vi "Lightfield Software.vi"() -> ()   [LabVIEW 2015]
doc: "Use this template to build a producer/consumer design pattern. Use this template when you need to execute a process, such as data analysis, when a data source, such as a triggered acquisition, produces data at an uneven rate and you need to execute the process when the data becomes available."
uses:
  etc/Other/Backups/Lightfield/Add-in and Automation SDK/Samples/LabVIEW Automation/lightfield-automation-labview/LightField Automation.lvclass
  <vilib>/Utility/file.llb/Write Delimited Spreadsheet (DBL).vi
  Documents/test/SDK 1.2.4 Installer/SDK 1.2.4 Installer/examples/Labview/win64/PE_Filter_SDK/PE_Filter_SDK.lvlib
panel:
  out "PLE total count":dbl
  out "LLTF error":errorcluster
  out "LLTF port":u32
  out "y_Count":dbl
  out "x_Count":dbl
  out "Time-counting":dbl
  in  "?":T1(tab)
  in  "PLE start":bool
  in  "PLE Pause":bool
  in  "PLE save":bool
  out "Min Wavelength":dbl
  out "Max Wavelength":dbl
  out "Current system":string
  out "PLE spectrum":dbl[][](graph)
  in  "Laser WL (nm)":dbl=450.0
  in  "Start WL":dbl=450.0
  in  "End WL":dbl=600.0
  in  "Step (nm)":dbl=1.0
  out "Current WL":dbl=450.0
  in  "Laser WL offset (nm)":dbl=-0.8
  in  "PLE_Autoscale intensity":bool
  in  "2D map_save":bool
  in  "2D map":bool
  in  "Step (um)":dbl=1.0
  in  "x_width (um)":dbl=10.0
  in  "y_width (um)":dbl=10.0
  out "Total Count":dbl
  in  "2D Pause":bool
  out "Cur_pos_x":dbl
  out "Cur_pos_y":dbl
  out "map_plot":dbl[][](graph)
  in  "WL Slide":cluster{dbl, dbl}(slide)={0.0, 1.4141414141414141} scale=700.8419246652234..738.7930212756685
  out "WL":dbl[](array[numeric])
  out "i_max":dbl
  out "i_min":dbl
  in  "Until when (s)":dbl=1.0 caption="Time Target (s)"
  in  "Time-series":bool
  out "Time-series graph":dbl[][](graph)
  in  "Times Pause":bool
  in  "Time Interval (s)":dbl=1.0 caption="Time Target (s)"
  in  "Time-series save":bool
  out "Runging time (s)":dbl
  out "map_data":dbl[][][](array[numeric])
  out "E727 error":errorcluster
  out "Min_y":dbl
  out "Min_x":dbl
  out "Max_y":dbl
  out "Max_x":dbl
  out "E727 Axes":string[](array[string])
  in  "USB settings":cluster{"S/N":string, "USB Search?":bool}={"S/N"="", "USB Search?"=TRUE}
  in  "E727":i32=1 min=1 step=1
  in  "Exposure Time (ms)":dbl=300.0
  in  "Centre WL (nm)":dbl=500.0
  out "Pixel Information":dbl[][](graph)
  in  "ROI":i32=1
  out "PL spectrum":T2(graph)
  out "LightField":refnum<class "LightField Automation.lvclass">
  in  "Experiment name":string="Exp"
  out "error out":errorcluster
  in  "Load":bool
  in  "Single Acquire":bool
  in  "stop":bool
  # "*If you selected \"Full sensor, Binned mode\" in ROI option at LightField, input \"1\""
  # "LLTF Control"
  # "LLTF Information"
  # "* The laser wavelength emitted from the LLTF is off-calibrated by around \"+0.8 nm\".\n* When you save the PLE data, All of the laser wavelength elements will be automatically added around [Laser WL offset \"+0.8 nm\"]."
  # "* Maximum of width is 100 um"
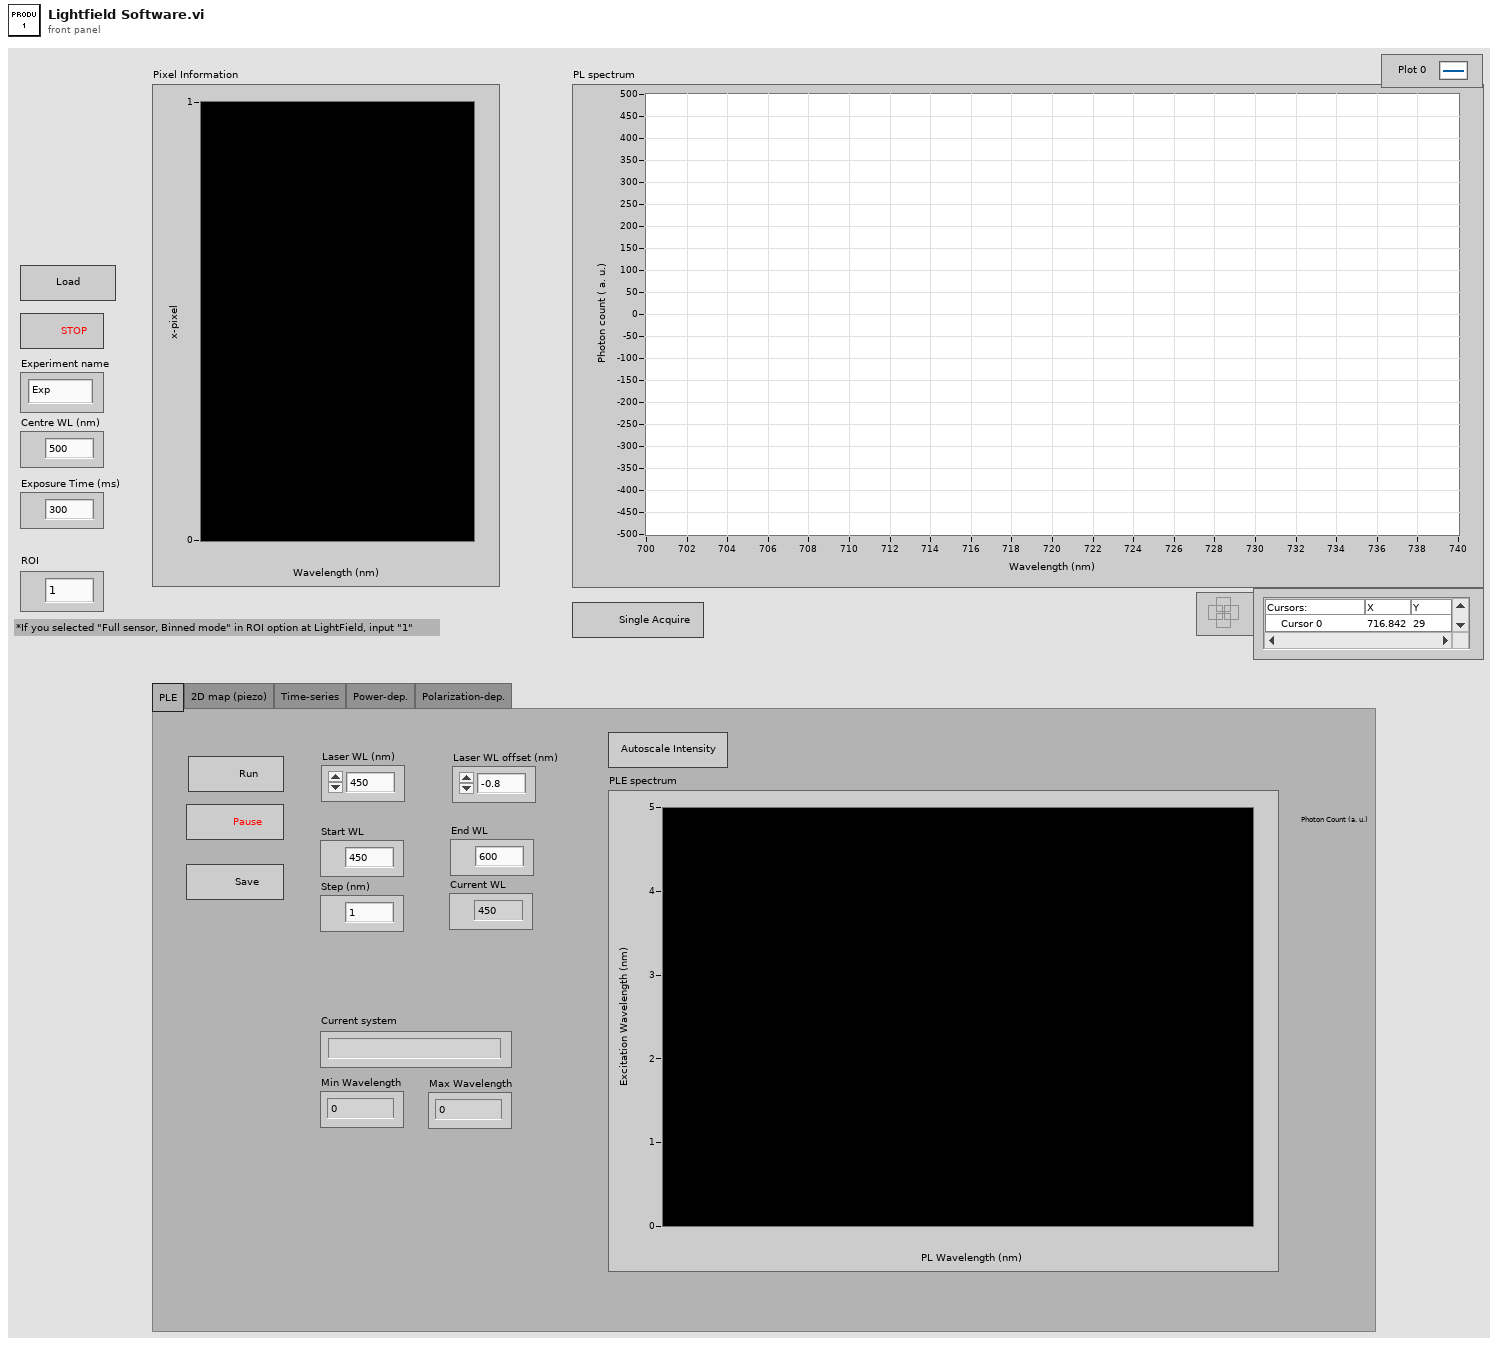
[diagram p1: front panel]
types:
  T1 = enum32{"PLE", "2D map (piezo)", "Time-series", "Power-dep.", "Polarization-dep."}
  T2 = cluster{"ColumnCalibration":dbl[], "ROI 1, Frame 1, Row 1":dbl[]}
  T3 = cluster{"Image":dbl[][][], "Frame Size":cluster{"F":i32, "Y":i32, "X":i32}}[]
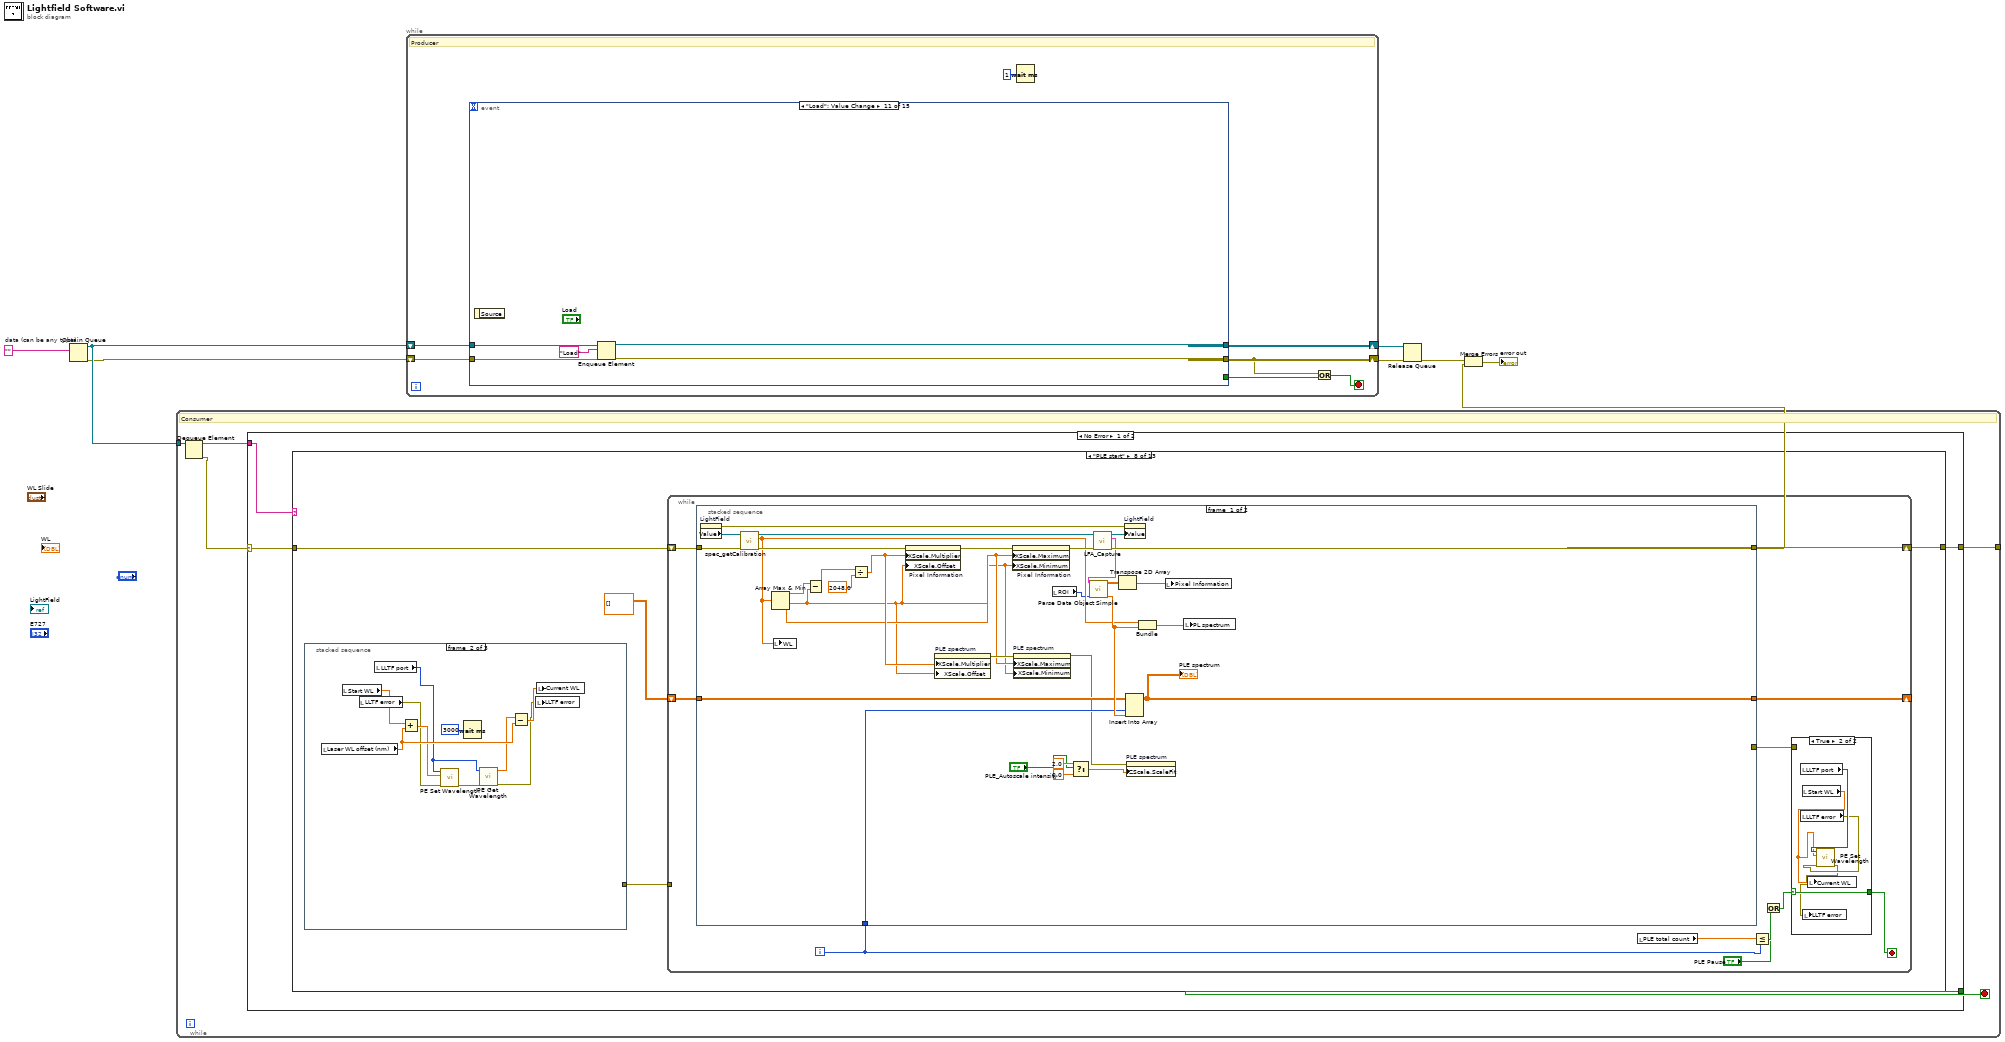
[diagram p0: block diagram]
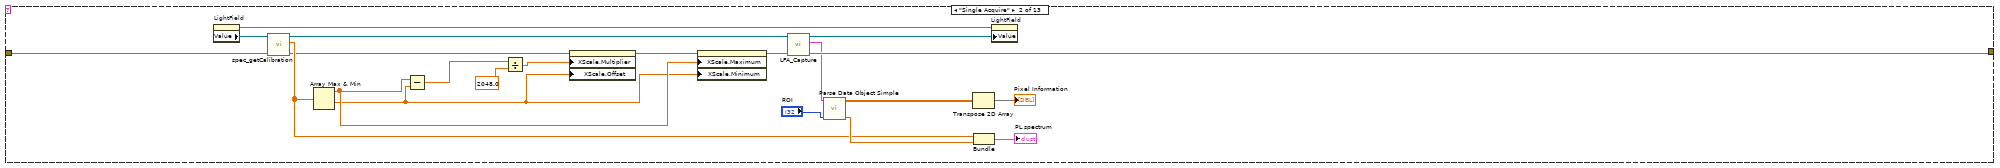
[diagram p3: hidden frame]
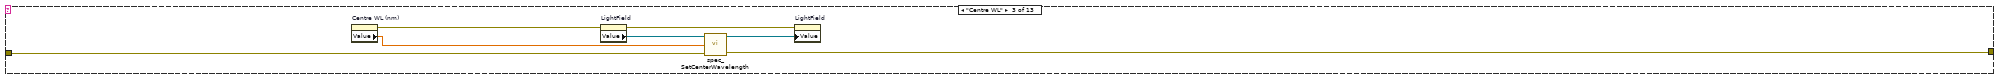
[diagram p4: hidden frame]
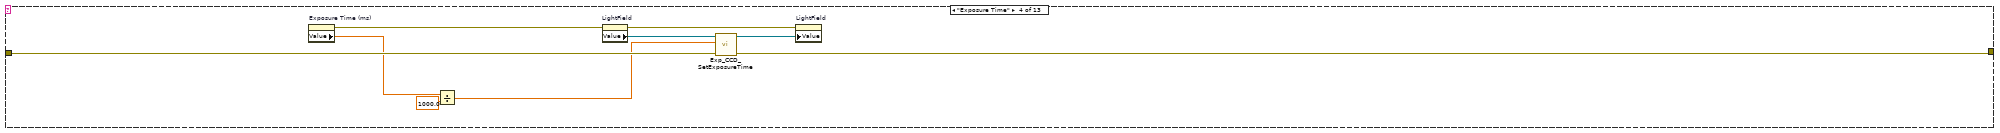
[diagram p5: hidden frame]
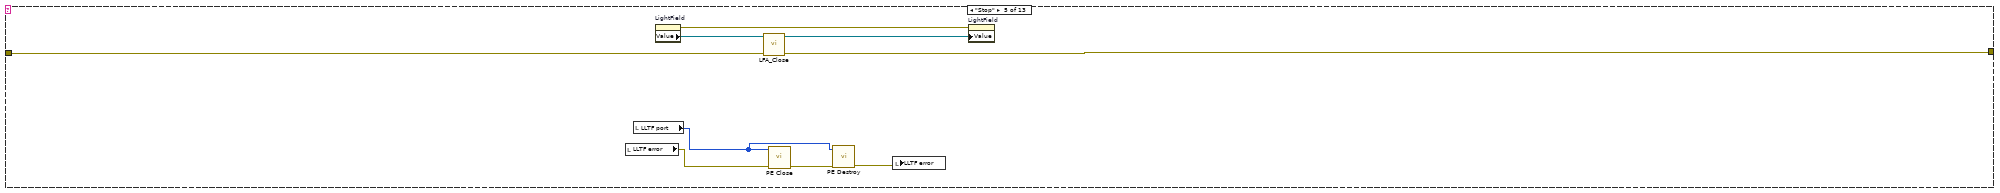
[diagram p6: hidden frame]
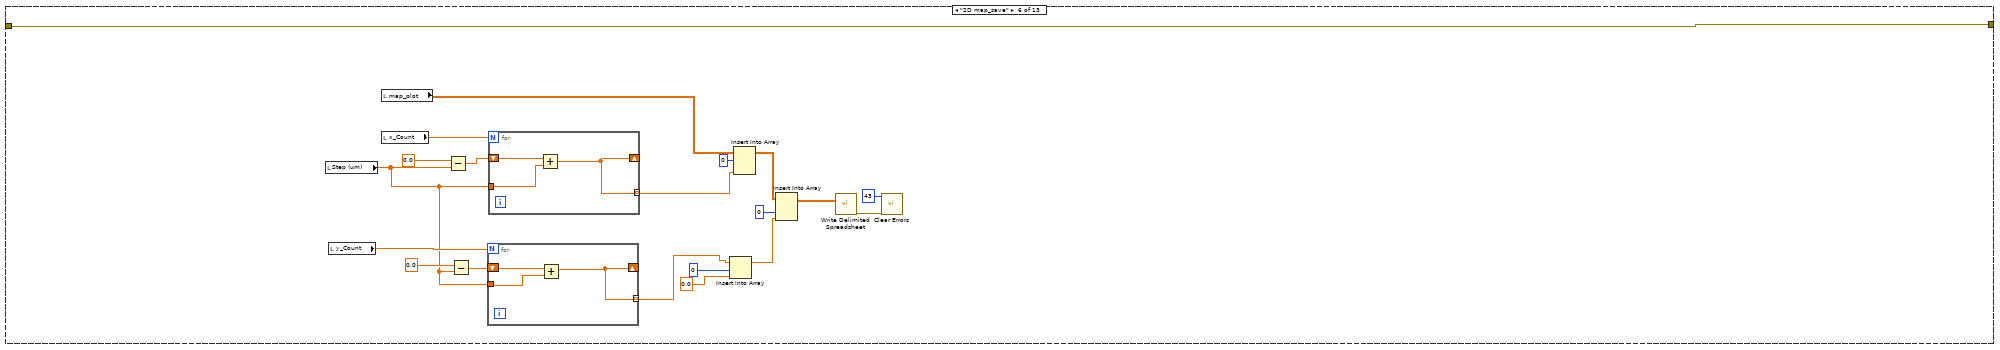
[diagram p7: hidden frame]
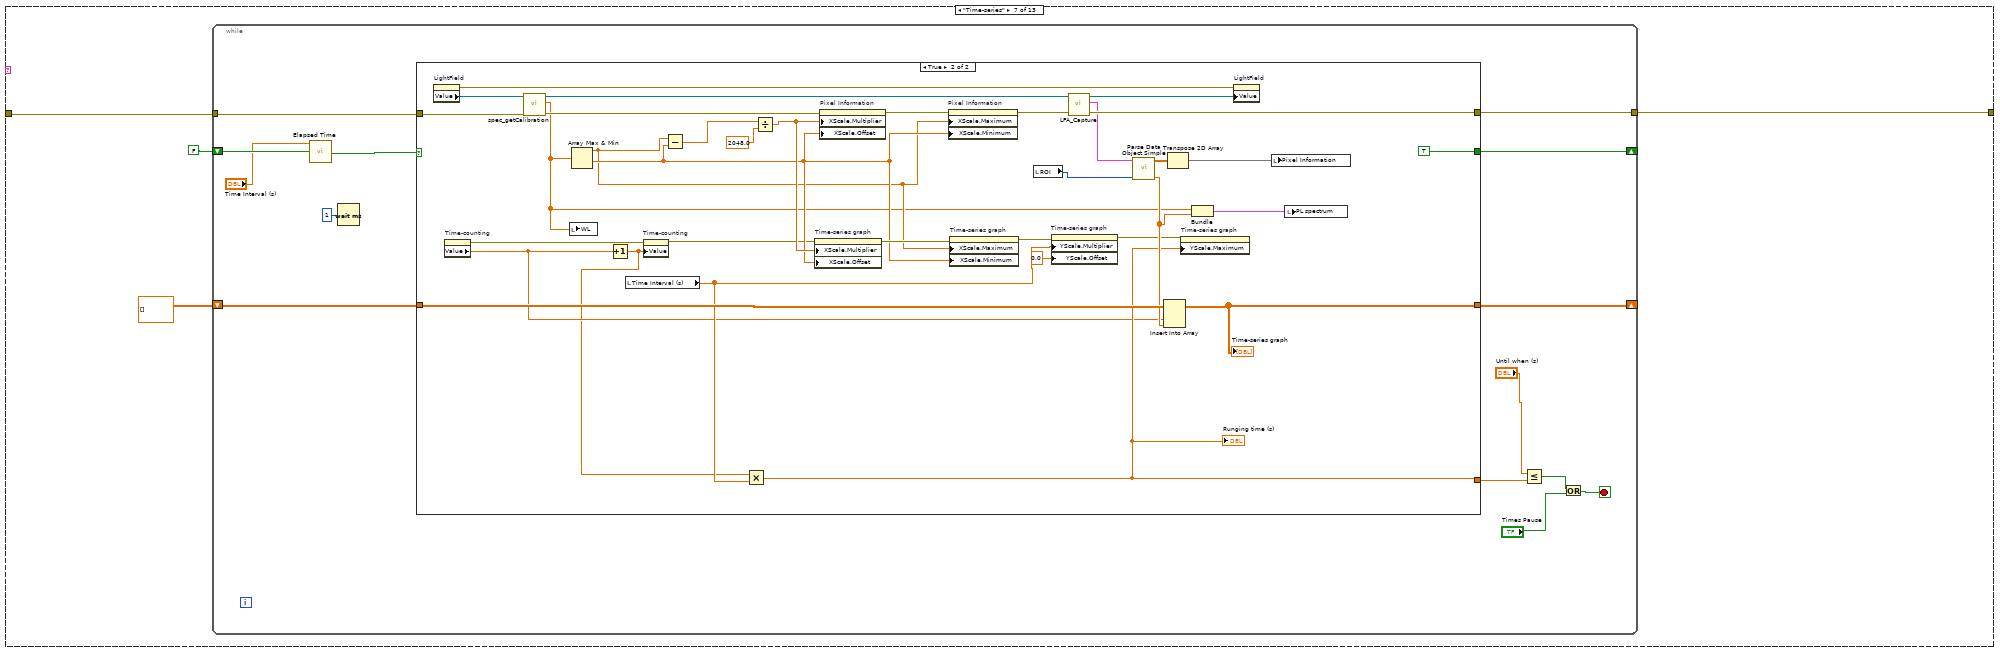
[diagram p8: hidden frame]
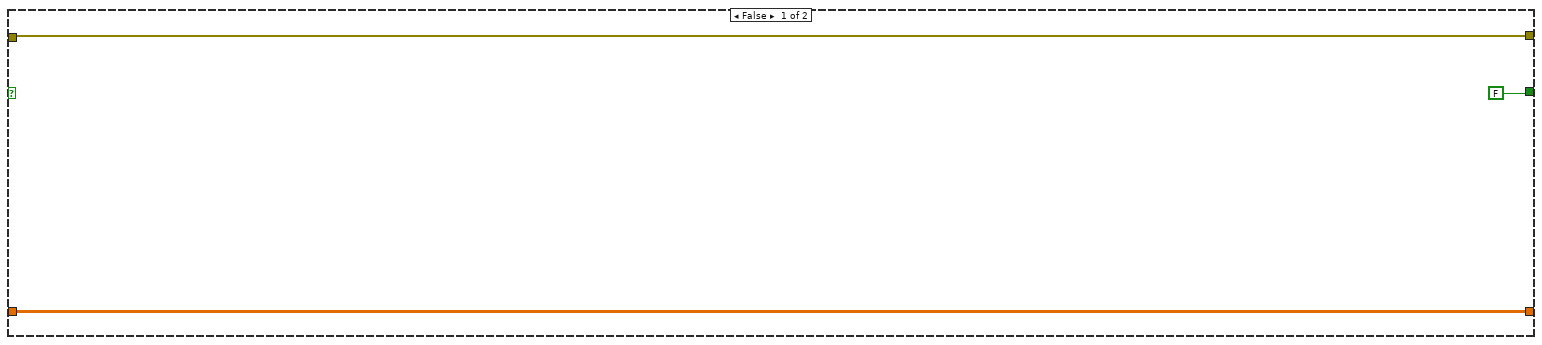
[diagram p9: hidden frame]
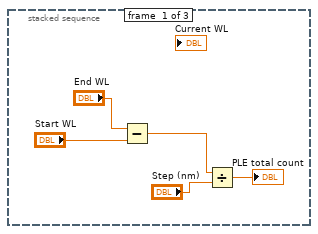
[diagram p10: hidden frame]
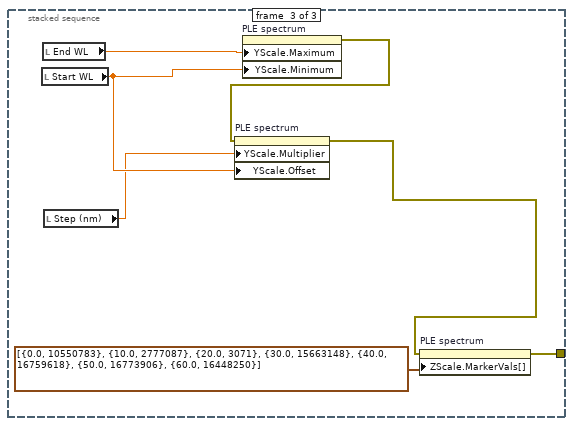
[diagram p11: hidden frame]
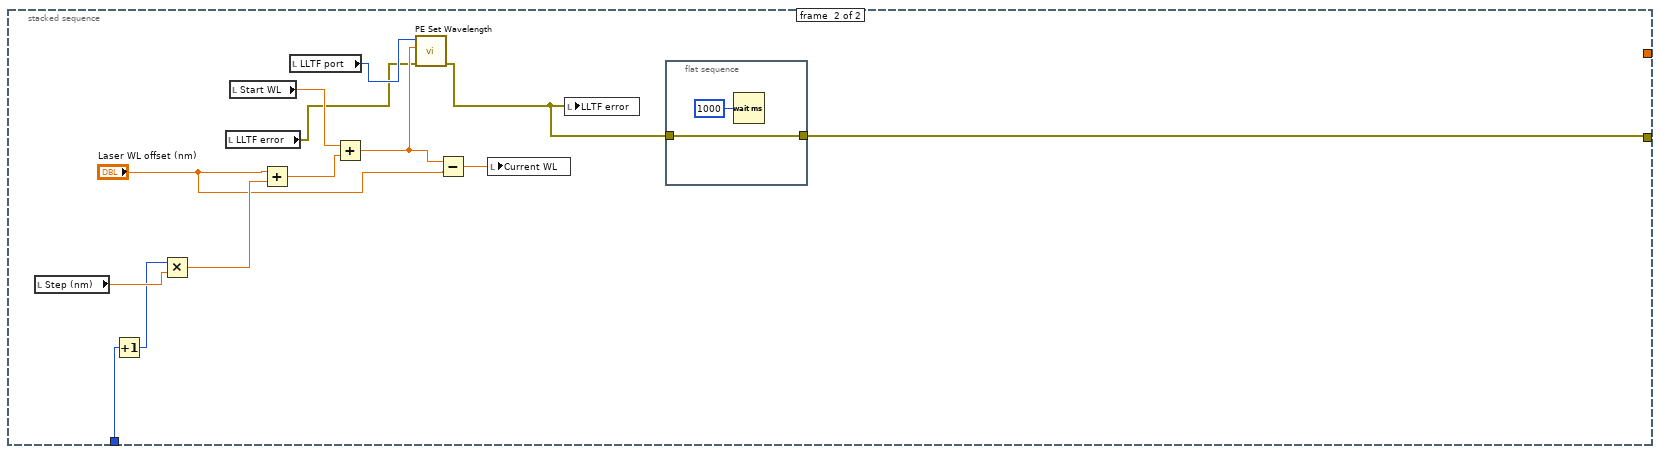
[diagram p13: hidden frame]
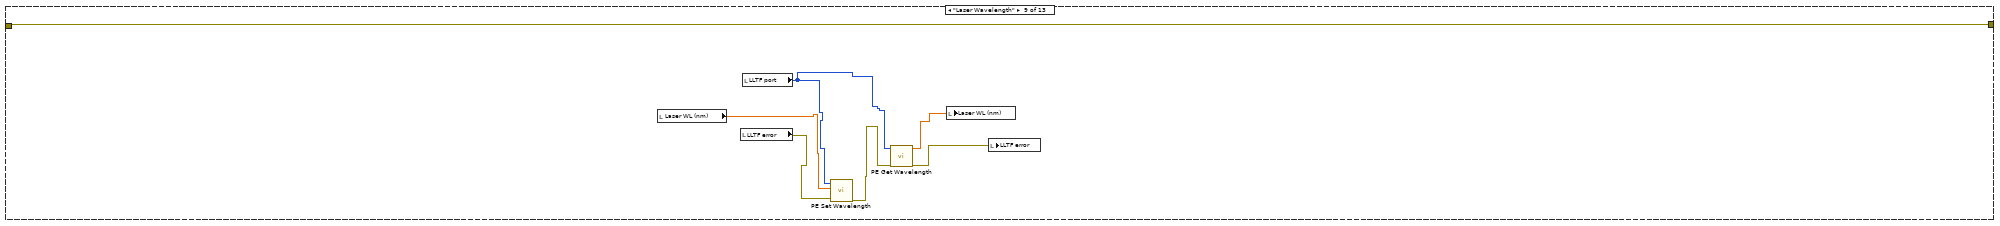
[diagram p14: hidden frame]
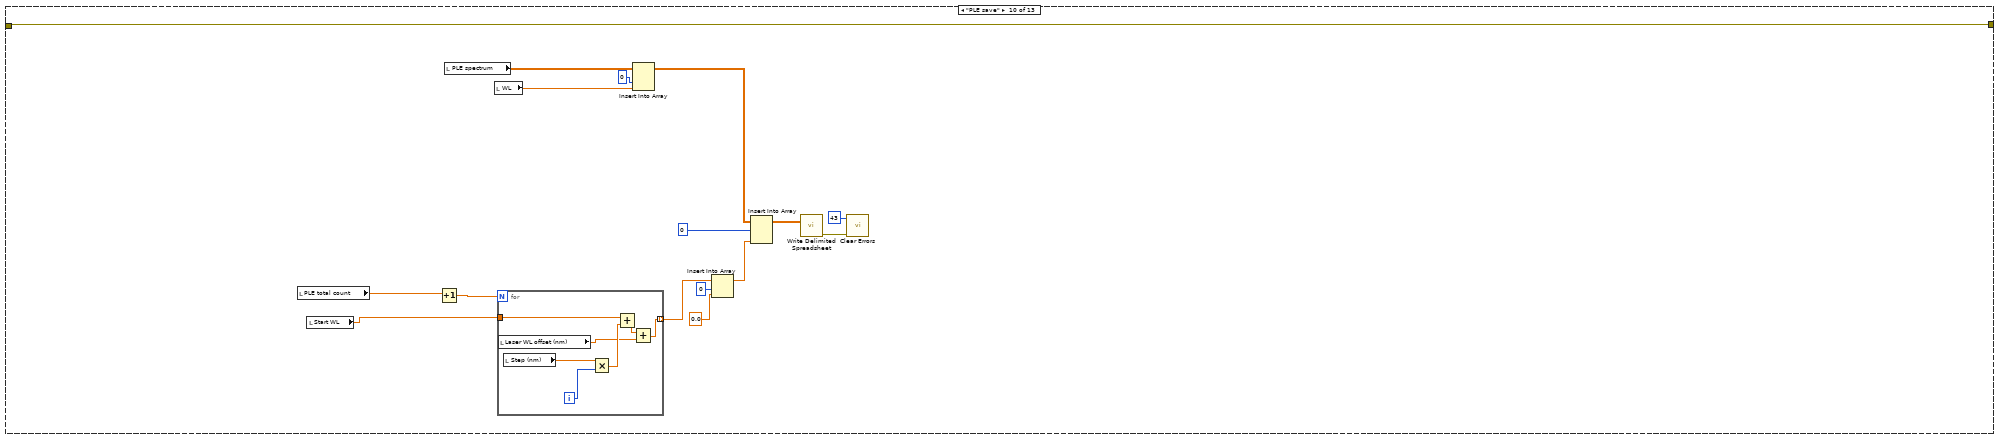
[diagram p15: hidden frame]
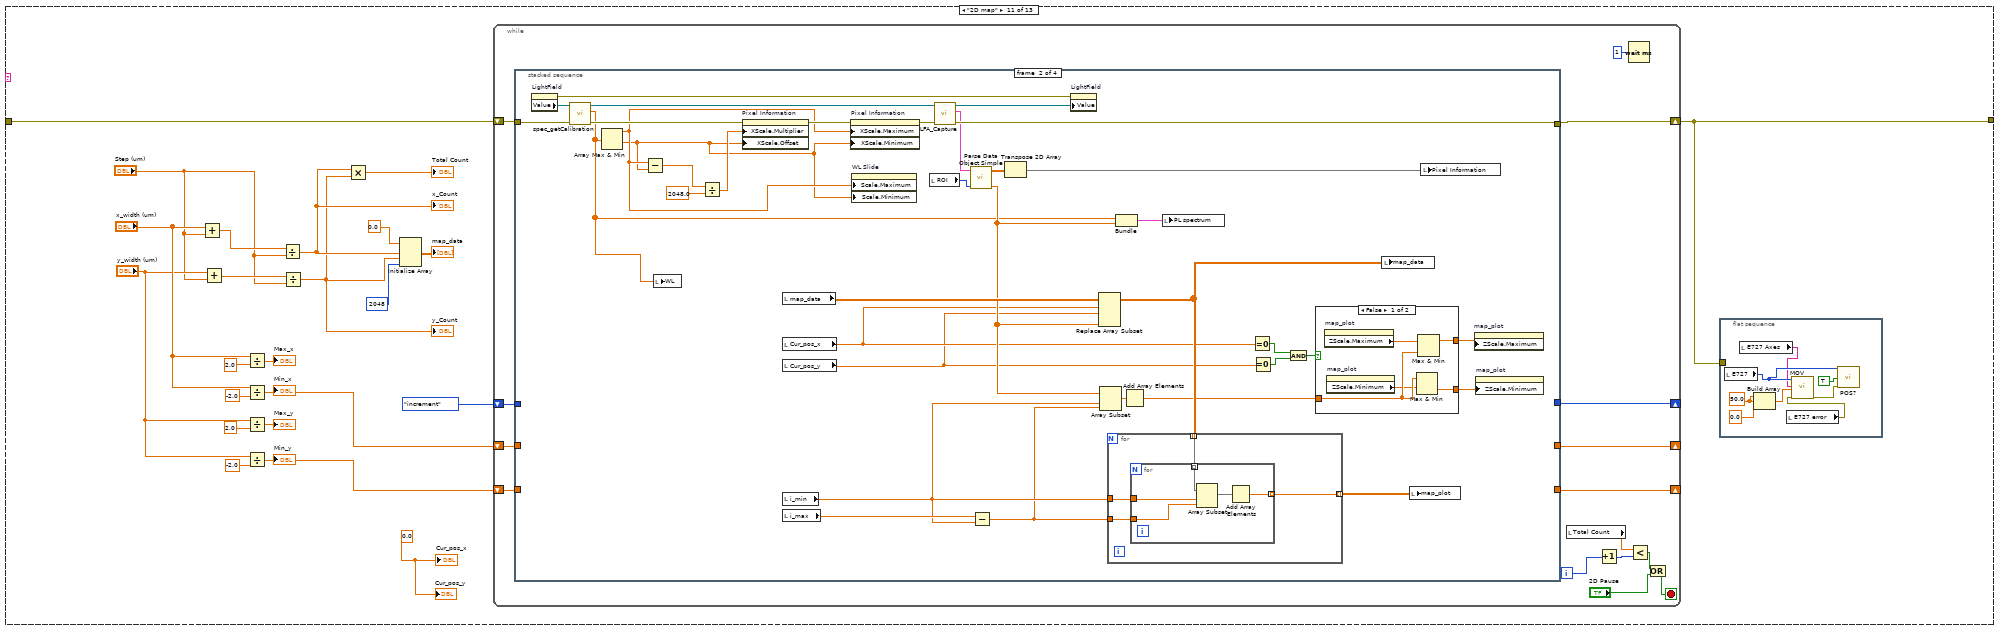
[diagram p16: hidden frame]
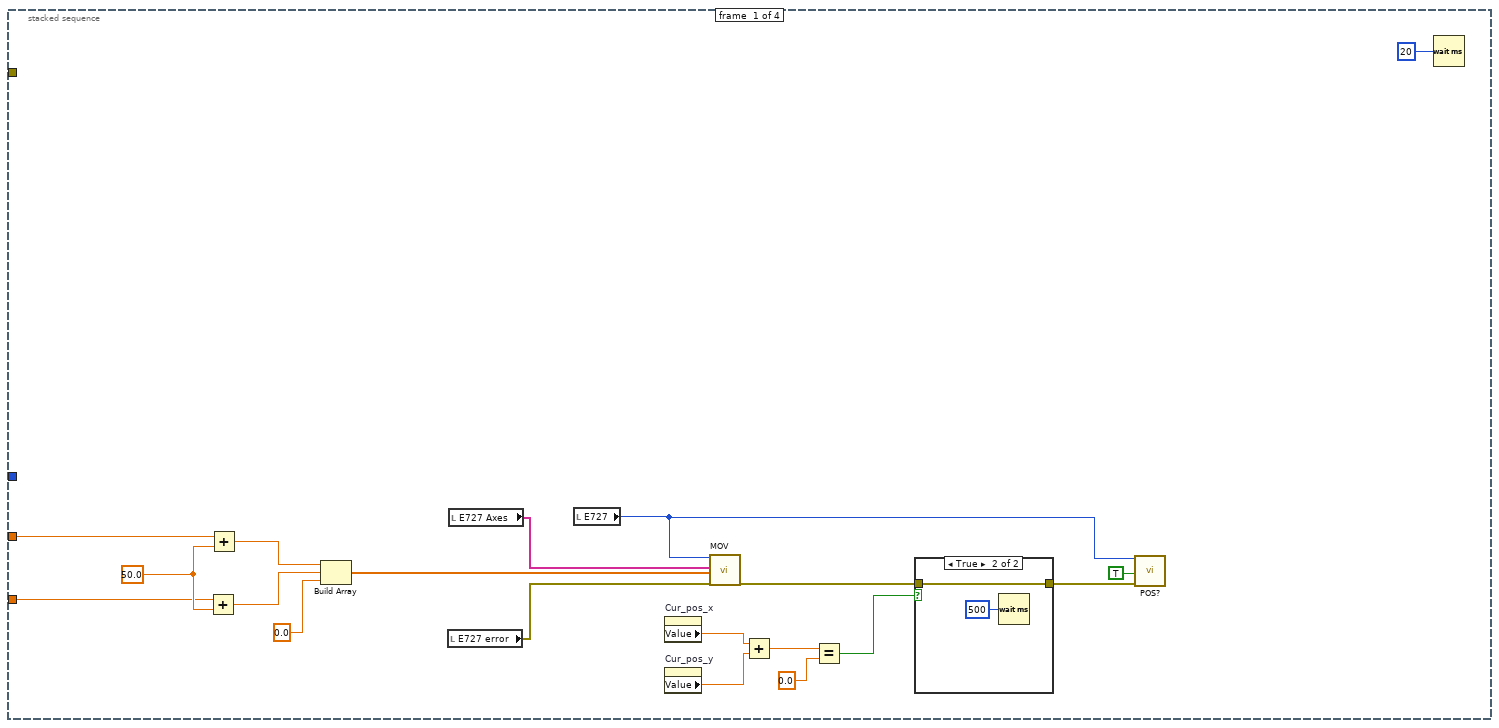
[diagram p17: hidden frame]
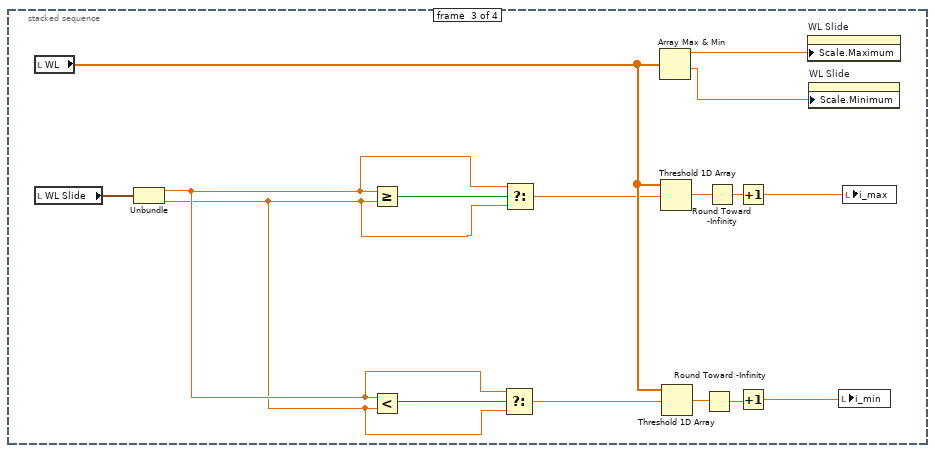
[diagram p20: hidden frame]
diagram:
  w4 = ""  # data (can be any type)
  n1 = Obtain Queue(element data type=w4) -> (queue out=w8:refnum<queue>, error out=w7:errorcluster)  [unwired: 4 in, 1 out]
  n2 = while {
    tunnel: w8 -> [w13]
    tunnel: [w9] -> w2
    stop <- w10 stop-if-true
    # "Consumer"
    n3 = Dequeue Element(queue=w13) -> (element=w11:string, error out=w12:errorcluster)  [unwired: 2 in, 2 out]
    n4 = case shown="No Error" w12 {
      selector: w12 -> [w15 w496]
      tunnel: w11 -> [w16 _]
      tunnel: [_ TRUE] -> w10
      tunnel: [w14 w496] -> w9
      frame No Error {
        n5 = case shown="\"PLE start\"" w16 {
          tunnel: w15 -> [w17 w26 w45 w54 w60 w75 w90 w148 w237 w253 w283 w463 w474]
          tunnel: [w17 w20 w44 w53 w59 w75 w91 w147 w237 w253 w261 w463 w480] -> w14
          frame "False", Default {
          }
          frame "Single Acquire" {
            n6 = property on="LightField" class="LVClassControl (strict)"() -> (error out=w24:errorcluster, "Value"=w25:refnum<class "LightField Automation.lvclass">)  [unwired: 2 in, 1 out]
            n7 = call "spec_getCalibration.vi"("error in (no error)"=w26, "LightField Automation in"=w25) -> ("error out"=w33:errorcluster, "ColumnCalibration"=w34:dbl[], "LightField Automation out"=w23:refnum<class "LightField Automation.lvclass">)  [unwired: 7 in]
            n8 = Array Max & Min(array=w34) -> (max value=w30:dbl, min value=w29:dbl)  [unwired: 2 out]
            n9 = Subtract(x=w30, y=w29) -> (x-y=w28:dbl)
            n10 = Divide(x=w28, y=2048.0) -> (x/y=w27:dbl)
            n11 = property on="Pixel Information" class="IntGraph (strict)"(error in=w33, "XScale.Multiplier"=w27, "XScale.Offset"=w29) -> (error out=w32:errorcluster)  [unwired: 1 in, 1 out]
            n12 = property on="Pixel Information" class="IntGraph (strict)"(error in=w32, "XScale.Maximum"=w30, "XScale.Minimum"=w29) -> (error out=w21:errorcluster)  [unwired: 1 in, 1 out]
            n13 = call "LFA_Capture.vi"("error in (no error)"=w21, "LightField Automation in"=w23) -> ("error out"=w20:errorcluster, "Data"=w19:T3, "LightField Automation out"=w22:refnum<class "LightField Automation.lvclass">)  [unwired: 7 in]
            n14 = call "Parse Data Object Simple.vi"("x"="ROI", "Data"=w19) -> ("ROI 1, Frame 1, Row 1"=w38:dbl[], "ROI 1, Frame 1"=w36:dbl[][])  [unwired: 8 in]
            n15 = Transpose 2D Array(2D array=w36) -> (transposed array=→"Pixel Information":dbl[][])
            n16 = Bundle("ColumnCalibration"=w34, "ROI 1, Frame 1, Row 1"=w38) -> (→"PL spectrum":T2)  [unwired: 1 in]
            n17 = property on="LightField" class="LVClassControl (strict)"(error in=w24, "Value"=w22) -> ()  [unwired: 1 in, 2 out]
          }
          frame "Centre WL" {
            n18 = property on="Centre WL (nm)" class="DigNum (strict)"() -> (error out=w39:errorcluster, "Value"=w40:dbl)  [unwired: 2 in, 1 out]
            n19 = property on="LightField" class="LVClassControl (strict)"(error in=w39) -> (error out=w42:errorcluster, "Value"=w43:refnum<class "LightField Automation.lvclass">)  [unwired: 1 in, 1 out]
            n20 = call "spec_SetCenterWavelength.vi"("error in (no error)"=w45, "Center Wavelength"=w40, "LightField Automation in"=w43) -> ("error out"=w44:errorcluster, "LightField Automation out"=w41:refnum<class "LightField Automation.lvclass">)  [unwired: 7 in]
            n21 = property on="LightField" class="LVClassControl (strict)"(error in=w42, "Value"=w41) -> ()  [unwired: 1 in, 2 out]
          }
          frame "Exposure Time" {
            n22 = property on="Exposure Time (ms)" class="DigNum (strict)"() -> (error out=w49:errorcluster, "Value"=w47:dbl)  [unwired: 2 in, 1 out]
            n23 = Divide(x=w47, y=1000.0) -> (x/y=w46:dbl)
            n24 = property on="LightField" class="LVClassControl (strict)"(error in=w49) -> (error out=w52:errorcluster, "Value"=w51:refnum<class "LightField Automation.lvclass">)  [unwired: 1 in, 1 out]
            n25 = call "Exp_CCD_SetExposureTime.vi"("error in (no error)"=w54, "Exposure Time (s)"=w46, "LightField Automation in"=w51) -> ("error out"=w53:errorcluster, "LightField Automation out"=w50:refnum<class "LightField Automation.lvclass">)  [unwired: 7 in]
            n26 = property on="LightField" class="LVClassControl (strict)"(error in=w52, "Value"=w50) -> ()  [unwired: 1 in, 2 out]
          }
          frame "Stop" {
            n27 = local read "LLTF error"() -> (w55:errorcluster)
            n28 = local read "LLTF port"() -> (w57:u32)
            n29 = property on="LightField" class="LVClassControl (strict)"() -> (error out=w63:errorcluster, "Value"=w62:refnum<class "LightField Automation.lvclass">)  [unwired: 2 in, 1 out]
            n30 = call "LFA_Close.vi"("error in (no error)"=w60, "LightField Automation in"=w62) -> ("error out"=w59:errorcluster, "LightField Automation out"=w61:refnum<class "LightField Automation.lvclass">)  [unwired: 8 in]
            n31 = call "PE Close.vi"("error in (no error)"=w55, "peHandle"=w57) -> ("error out"=w56:errorcluster)  [unwired: 9 in]
            n32 = call "PE Destroy.vi"("error in (no error)"=w56, "peHandle"=w57) -> ("error out"=w58:errorcluster)  [unwired: 9 in]
            n33 = local write "LLTF error"(w58) -> ()
            n34 = property on="LightField" class="LVClassControl (strict)"(error in=w63, "Value"=w61) -> ()  [unwired: 1 in, 2 out]
          }
          frame "2D map_save" {
            n35 = local read "Step (um)"() -> (w68:dbl)
            n36 = local read "y_Count"() -> (w82:dbl)
            n37 = local read "map_plot"() -> (w81:dbl[][])
            n38 = local read "x_Count"() -> (w83:dbl)
            n39 = Subtract(x=0.0, y=w68) -> (x-y=w71:dbl)
            n40 = Subtract(x=0.0, y=w68) -> (x-y=w69:dbl)
            n41 = for {
              N: w82 -> [_]
              tunnel: [w84] -> w66 mode=indexing
              shift-right: [w84] -> _
              shift-left: w69 -> [w86]
              tunnel: w68 -> [w85]
              n42 = Add(x=w86, y=w85) -> (x+y=w84:dbl)
            }
            n43 = for {
              N: w83 -> [_]
              tunnel: [w88] -> w73 mode=indexing
              shift-right: [w88] -> _
              shift-left: w71 -> [w89]
              tunnel: w68 -> [w87]
              n44 = Add(x=w89, y=w87) -> (x+y=w88:dbl)
            }
            n45 = Insert Into Array(array=w66, index=0, new element=0.0 ("new element/subarray")) -> (w64:dbl[])
            n46 = Insert Into Array(array=w81, index (row)=0, new element=w73) -> (w79:dbl[][])  [unwired: 1 in]
            n47 = Insert Into Array(array=w79, index (col)=0 ("index (row)"), new element=w64) -> (w78:dbl[][])  [unwired: 1 in]
            n48 = call-poly <vilib>:"Write Delimited Spreadsheet.vi"("2D data"=w78) -> ("error out"=w77:errorcluster)  [unwired: 13 in, 1 out]
            n49 = call <vilib>:"Clear Errors.vi"("error in (no error)"=w77, "specific error code to clear (0: all)"=43) -> ()  [unwired: 4 in, 2 out]
          }
          frame "Time-series" {
            n50 = while {
              shift-right: [w105] -> _
              shift-left: FALSE -> [w107]
              shift-right: [w101] -> _
              shift-left: dbl[][] [] -> [w102]
              tunnel: [w100] -> w91
              tunnel: w90 -> [w99]
              stop <- w96 stop-if-true
              n51 = call "Elapsed Time"("Time Target (s)"="Time Interval (s)", "Reset"=w107) -> ("Time has Elapsed"=w106:bool)  [unwired: 10 in, 7 out]
              n52 = Wait (ms)(milliseconds to wait=u32 1) -> ()  [unwired: 1 out]
              n53 = case shown="True" w106 {
                tunnel: [FALSE TRUE] -> w105
                tunnel: w102 -> [w109 w134]
                tunnel: [w109 w126] -> w101
                tunnel: [w108 w114] -> w100
                tunnel: w99 -> [w108 w129]
                tunnel: [_ w124] -> w95
                frame False {
                }
                frame True {
                  n54 = property on="LightField" class="LVClassControl (strict)"() -> (error out=w137:errorcluster, "Value"=w136:refnum<class "LightField Automation.lvclass">)  [unwired: 2 in, 1 out]
                  n55 = property on="Time-counting" class="DigNum (strict)"() -> (error out=w128:errorcluster, "Value"=w119:dbl)  [unwired: 2 in, 1 out]
                  n56 = call "spec_getCalibration.vi"("error in (no error)"=w129, "LightField Automation in"=w136) -> ("error out"=w141:errorcluster, "ColumnCalibration"=w112:dbl[], "LightField Automation out"=w117:refnum<class "LightField Automation.lvclass">)  [unwired: 7 in]
                  n57 = local write "WL"(w112) -> ()
                  n58 = Array Max & Min(array=w112) -> (max value=w130:dbl, min value=w131:dbl)  [unwired: 2 out]
                  n59 = Increment(x=w119) -> (x+1=w118:dbl)
                  n60 = local read "Time Interval (s)"() -> (w120:dbl)
                  n61 = property on="Time-counting" class="DigNum (strict)"(error in=w128, "Value"=w118) -> (error out=w125:errorcluster)  [unwired: 1 in, 1 out]
                  n62 = Subtract(x=w130, y=w131) -> (x-y=w140:dbl)
                  n63 = Multiply(x=w118, y=w120) -> (x*y=w124:dbl)
                  "Runging time (s)" <- w124
                  n64 = Divide(x=w140, y=2048.0) -> (x/y=w133:dbl)
                  n65 = property on="Time-series graph" class="IntGraph (strict)"(error in=w125, "XScale.Multiplier"=w133, "XScale.Offset"=w131) -> (error out=w132:errorcluster)  [unwired: 1 in, 1 out]
                  n66 = property on="Pixel Information" class="IntGraph (strict)"(error in=w141, "XScale.Multiplier"=w133, "XScale.Offset"=w131) -> (error out=w139:errorcluster)  [unwired: 1 in, 1 out]
                  n67 = property on="Pixel Information" class="IntGraph (strict)"(error in=w139, "XScale.Maximum"=w130, "XScale.Minimum"=w131) -> (error out=w115:errorcluster)  [unwired: 1 in, 1 out]
                  n68 = property on="Time-series graph" class="IntGraph (strict)"(error in=w132, "XScale.Maximum"=w130, "XScale.Minimum"=w131) -> (error out=w123:errorcluster)  [unwired: 1 in, 1 out]
                  n69 = local read "ROI"() -> (w111:i32)
                  n70 = property on="Time-series graph" class="IntGraph (strict)"(error in=w123, "YScale.Multiplier"=w120, "YScale.Offset"=0.0 ("Y Scale.Offset and Multiplier:Offset")) -> (error out=w122:errorcluster)  [unwired: 1 in, 1 out]
                  n71 = call "LFA_Capture.vi"("error in (no error)"=w115, "LightField Automation in"=w117) -> ("error out"=w114:errorcluster, "Data"=w113:T3, "LightField Automation out"=w116:refnum<class "LightField Automation.lvclass">)  [unwired: 7 in]
                  n72 = call "Parse Data Object Simple.vi"("x"=w111, "Data"=w113) -> ("ROI 1, Frame 1, Row 1"=w127:dbl[], "ROI 1, Frame 1"=w138:dbl[][])  [unwired: 8 in]
                  n73 = Insert Into Array(array=w134, index (col)=w119, new element=w127) -> (w126:dbl[][])  [unwired: 1 in]
                  "Time-series graph" <- w126
                  n74 = Transpose 2D Array(2D array=w138) -> (transposed array=w142:dbl[][])
                  n75 = property on="Time-series graph" class="IntGraph (strict)"(error in=w122, "YScale.Maximum"=w124) -> ()  [unwired: 1 in, 2 out]
                  n76 = Bundle("ColumnCalibration"=w112, "ROI 1, Frame 1, Row 1"=w127) -> (w143:T2)  [unwired: 1 in]
                  n77 = property on="LightField" class="LVClassControl (strict)"(error in=w137, "Value"=w116) -> ()  [unwired: 1 in, 2 out]
                  n78 = local write "Pixel Information"(w142) -> ()
                  n79 = local write "PL spectrum"(w143) -> ()
                }
              }
              n80 = Less Or Equal?(x="Until when (s)", y=w95) -> (x <= y?=w98:bool)
              n81 = Or(x=w98, y="Times Pause") -> (x .or. y?=w96:bool)
            }
          }
          frame "PLE start" {
            n82 = stacked-sequence {
              tunnel: [_ _ w168] -> w145
              frame #0 {
                n83 = Subtract(x="End WL", y="Start WL") -> (x-y=w151:dbl)
                n84 = Divide(x=w151, y="Step (nm)") -> (x/y=→"PLE total count":dbl)
              }
              frame #1 {
                n85 = local read "Laser WL offset (nm)"() -> (w161:dbl)
                n86 = local read "Start WL"() -> (w162:dbl)
                n87 = local read "LLTF error"() -> (w155:errorcluster)
                n88 = local read "LLTF port"() -> (w154:u32)
                n89 = Add(x=w162, y=w161) -> (x+y=w156:dbl)
                n90 = call "PE Set Wavelength.vi"("error in (no error)"=w155, "wavelength"=w156, "peHandle"=w154) -> ("error out"=w159:errorcluster)  [unwired: 8 in]
                n91 = Wait (ms)(milliseconds to wait=u32 3000) -> ()  [unwired: 1 out]
                n92 = call "PE Get Wavelength.vi"("error in (no error)"=w159, "peHandle"=w154) -> ("error out"=w158:errorcluster, "wavelength"=w157:dbl)  [unwired: 8 in]
                n93 = Subtract(x=w157, y=w161) -> (x-y=w160:dbl)
                n94 = local write "LLTF error"(w158) -> ()
                n95 = local write "Current WL"(w160) -> ()
              }
              frame #2 {
                n96 = local read "Start WL"() -> (w167:dbl)
                n97 = local read "End WL"() -> (w169:dbl)
                n98 = local read "Step (nm)"() -> (w166:dbl)
                n99 = property on="PLE spectrum" class="IntGraph (strict)"("YScale.Maximum"=w169, "YScale.Minimum"=w167) -> (error out=w165:errorcluster)  [unwired: 2 in, 1 out]
                n100 = property on="PLE spectrum" class="IntGraph (strict)"(error in=w165, "YScale.Multiplier"=w166, "YScale.Offset"=w167) -> (error out=w164:errorcluster)  [unwired: 1 in, 1 out]
                n101 = property on="PLE spectrum" class="IntGraph (strict)"(error in=w164, "ZScale.MarkerVals[]"=cluster{dbl, u32}[] [{0.0, 10550783}, {10.0, 2777087}, {20.0, 3071}, {30.0, 15663148}, {40.0, 16759618}, {50.0, 16773906}, {60.0, 16448250}] ("Z Scale.Marker Values[]")) -> (error out=w168:errorcluster)  [unwired: 1 in, 1 out]
              }
            }
            n102 = while {
              shift-right: [w179] -> w147
              shift-left: w148 -> [w180]
              shift-right: [w177] -> _
              shift-left: dbl[][] [] -> [w178]
              tunnel: w145 -> [_]
              i -> [w173]
              stop <- w172 stop-if-true
              n103 = stacked-sequence {
                tunnel: w180 -> [w215 _]
                tunnel: [w214 _] -> w179
                tunnel: w178 -> [w199 _]
                tunnel: [w198 _] -> w177
                tunnel: w173 -> [w197 w227]
                tunnel: [_ w220] -> w171
                frame #0 {
                  n104 = property on="LightField" class="LVClassControl (strict)"() -> (error out=w210:errorcluster, "Value"=w212:refnum<class "LightField Automation.lvclass">)  [unwired: 2 in, 1 out]
                  n105 = call "spec_getCalibration.vi"("error in (no error)"=w215, "LightField Automation in"=w212) -> ("error out"=w203:errorcluster, "ColumnCalibration"=w192:dbl[], "LightField Automation out"=w213:refnum<class "LightField Automation.lvclass">)  [unwired: 7 in]
                  n106 = Array Max & Min(array=w192) -> (max value=w194:dbl, min value=w193:dbl)  [unwired: 2 out]
                  n107 = local write "WL"(w192) -> ()
                  n108 = Subtract(x=w194, y=w193) -> (x-y=w204:dbl)
                  n109 = Divide(x=w204, y=2048.0) -> (x/y=w195:dbl)
                  n110 = property on="Pixel Information" class="IntGraph (strict)"(error in=w203, "XScale.Multiplier"=w195, "XScale.Offset"=w193) -> (error out=w202:errorcluster)  [unwired: 1 in, 1 out]
                  n111 = property on="PLE spectrum" class="IntGraph (strict)"("XScale.Multiplier"=w195, "XScale.Offset"=w193) -> (error out=w196:errorcluster)  [unwired: 2 in, 1 out]
                  n112 = property on="Pixel Information" class="IntGraph (strict)"(error in=w202, "XScale.Maximum"=w194, "XScale.Minimum"=w193) -> (error out=w201:errorcluster)  [unwired: 1 in, 1 out]
                  n113 = property on="PLE spectrum" class="IntGraph (strict)"(error in=w196, "XScale.Maximum"=w194, "XScale.Minimum"=w193) -> (error out=w191:errorcluster)  [unwired: 1 in, 1 out]
                  n114 = local read "ROI"() -> (w186:i32)
                  n115 = Select(t=2.0, s="PLE_Autoscale intensity", f=0.0) -> (s? t:f=w190:dbl)
                  n116 = call "LFA_Capture.vi"("error in (no error)"=w201, "LightField Automation in"=w213) -> ("error out"=w214:errorcluster, "Data"=w208:T3, "LightField Automation out"=w211:refnum<class "LightField Automation.lvclass">)  [unwired: 7 in]
                  n117 = call "Parse Data Object Simple.vi"("x"=w186, "Data"=w208) -> ("ROI 1, Frame 1, Row 1"=w200:dbl[], "ROI 1, Frame 1"=w209:dbl[][])  [unwired: 8 in]
                  n118 = Transpose 2D Array(2D array=w209) -> (transposed array=w206:dbl[][])
                  n119 = property on="LightField" class="LVClassControl (strict)"(error in=w210, "Value"=w211) -> ()  [unwired: 1 in, 2 out]
                  n120 = Insert Into Array(array=w199, index (col)=w197, new element=w200) -> (w198:dbl[][])  [unwired: 1 in]
                  "PLE spectrum" <- w198
                  n121 = property on="PLE spectrum" class="IntGraph (strict)"(error in=w191, "ZScale.ScaleFit"=w190) -> ()  [unwired: 1 in, 2 out]
                  n122 = Bundle("ColumnCalibration"=w192, "ROI 1, Frame 1, Row 1"=w200) -> (w207:T2)  [unwired: 1 in]
                  n123 = local write "Pixel Information"(w206) -> ()
                  n124 = local write "PL spectrum"(w207) -> ()
                }
                frame #1 {
                  n125 = local read "Step (nm)"() -> (w228:dbl)
                  n126 = Increment(x=w227) -> (x+1=w226:i32)
                  n127 = Multiply(x=w226, y=w228) -> (x*y=w223:dbl)
                  n128 = local read "LLTF error"() -> (w217:errorcluster)
                  n129 = local read "Start WL"() -> (w225:dbl)
                  n130 = Add(x="Laser WL offset (nm)", y=w223) -> (x+y=w224:dbl)
                  n131 = local read "LLTF port"() -> (w219:u32)
                  n132 = Add(x=w225, y=w224) -> (x+y=w218:dbl)
                  n133 = call "PE Set Wavelength.vi"("error in (no error)"=w217, "wavelength"=w218, "peHandle"=w219) -> ("error out"=w216:errorcluster)  [unwired: 8 in]
                  n134 = Subtract(x=w218, y="Laser WL offset (nm)") -> (x-y=w221:dbl)
                  n135 = local write "Current WL"(w221) -> ()
                  n136 = local write "LLTF error"(w216) -> ()
                  n137 = flat-sequence {
                    tunnel: w216 -> [w229]
                    tunnel: [w229] -> w220
                    frame #0 {
                      n138 = Wait (ms)(milliseconds to wait=u32 1000) -> ()  [unwired: 1 out]
                    }
                  }
                }
              }
              n139 = local read "PLE total count"() -> (w175:dbl)
              n140 = Less Or Equal?(x=w175, y=w173) -> (x <= y?=w176:bool)
              n141 = Or(x=w176, y="PLE Pause") -> (x .or. y?=w172:bool)
              n142 = case shown="True" w172 {
                selector: w172 -> [_ w185]
                tunnel: [_ w185] -> _
                tunnel: w171 -> [_ _]
                frame False {
                }
                frame True {
                  n143 = local read "LLTF port"() -> (w184:u32)
                  n144 = local read "LLTF error"() -> (w182:errorcluster)
                  n145 = local read "Start WL"() -> (w183:dbl)
                  n146 = local write "Current WL"(w183) -> ()
                  n147 = call "PE Set Wavelength.vi"("error in (no error)"=w182, "wavelength"=w183, "peHandle"=w184) -> ("error out"=w181:errorcluster)  [unwired: 8 in]
                  n148 = local write "LLTF error"(w181) -> ()
                }
              }
            }
          }
          frame "Laser Wavelength" {
            n149 = local read "Laser WL (nm)"() -> (w236:dbl)
            n150 = local read "LLTF error"() -> (w235:errorcluster)
            n151 = local read "LLTF port"() -> (w234:u32)
            n152 = call "PE Set Wavelength.vi"("error in (no error)"=w235, "wavelength"=w236, "peHandle"=w234) -> ("error out"=w233:errorcluster)  [unwired: 8 in]
            n153 = call "PE Get Wavelength.vi"("error in (no error)"=w233, "peHandle"=w234) -> ("error out"=w232:errorcluster, "wavelength"=w231:dbl)  [unwired: 8 in]
            n154 = local write "Laser WL (nm)"(w231) -> ()
            n155 = local write "LLTF error"(w232) -> ()
          }
          frame "PLE save" {
            n156 = local read "PLE total count"() -> (w239:dbl)
            n157 = local read "Start WL"() -> (w240:dbl)
            n158 = Increment(x=w239) -> (x+1=w238:dbl)
            n159 = local read "PLE spectrum"() -> (w242:dbl[][])
            n160 = local read "WL"() -> (w241:dbl[])
            n161 = for {
              N: w238 -> [_]
              tunnel: [w254] -> w245 mode=indexing
              tunnel: w240 -> [w260]
              i -> [w258]
              n162 = local read "Laser WL offset (nm)"() -> (w255:dbl)
              n163 = local read "Step (nm)"() -> (w259:dbl)
              n164 = Multiply(x=w259, y=w258) -> (x*y=w257:dbl)
              n165 = Add(x=w260, y=w257) -> (x+y=w256:dbl)
              n166 = Add(x=w256, y=w255) -> (x+y=w254:dbl)
            }
            n167 = Insert Into Array(array=w242, index (col)=0 ("index (row)"), new element=w241) -> (w249:dbl[][])  [unwired: 1 in]
            n168 = Insert Into Array(array=w245, index=0, new element=0.0 ("new element/subarray")) -> (w244:dbl[])
            n169 = Insert Into Array(array=w249, index (row)=0 ("disabled index (col)"), new element=w244) -> (w250:dbl[][])  [unwired: 1 in]
            n170 = call-poly <vilib>:"Write Delimited Spreadsheet.vi"("2D data"=w250) -> ("error out"=w252:errorcluster)  [unwired: 13 in, 1 out]
            n171 = call <vilib>:"Clear Errors.vi"("error in (no error)"=w252, "specific error code to clear (0: all)"=43) -> ()  [unwired: 4 in, 2 out]
          }
          frame "2D map" {
            w270 = 0.0 ("y_width (um) 2")
            n172 = Add(x="x_width (um)", y="Step (um)") -> (x+y=w268:dbl)
            n173 = Add(x="y_width (um)", y="Step (um)") -> (x+y=w266:dbl)
            n174 = Divide(x="x_width (um)", y=2.0) -> (x/y=→"Max_x":dbl)
            n175 = Divide(x="x_width (um)", y=-2.0) -> (x/y=w275:dbl)
            "Min_x" <- w275
            n176 = Divide(x="y_width (um)", y=2.0) -> (x/y=→"Max_y":dbl)
            n177 = Divide(x="y_width (um)", y=-2.0) -> (x/y=w276:dbl)
            "Min_y" <- w276
            n178 = Divide(x=w268, y="Step (um)") -> (x/y=w264:dbl)
            "x_Count" <- w264
            n179 = Divide(x=w266, y="Step (um)") -> (x/y=w263:dbl)
            "y_Count" <- w263
            n180 = Multiply(x=w264, y=w263) -> (x*y=→"Total Count":dbl)
            n181 = Initialize Array(0.0 ("element"), w264, w263, 2048 ("dimension size")) -> (→"map_data":dbl[][][])
            n182 = while {
              shift-right: [w299] -> w261
              shift-left: w283 -> [w300]
              shift-right: [w306] -> _
              shift-left: w275 -> [w302]
              shift-right: [w305] -> _
              shift-left: w276 -> [w301]
              shift-right: [w303] -> _
              shift-left: enum16{"decrement", "increment"}."increment" ("Enum") -> [w304]
              i -> [w292]
              stop <- w293 stop-if-true
              n183 = stacked-sequence {
                tunnel: [_ _ _ w397] -> w306
                tunnel: [_ _ _ w396] -> w305
                tunnel: w304 -> [_ _ _ w401]
                tunnel: [_ _ _ w398] -> w303
                tunnel: w302 -> [w321 _ _ w400]
                tunnel: w301 -> [w320 _ _ w399]
                tunnel: w300 -> [_ w355 _ _]
                tunnel: [_ w332 _ _] -> w299
                frame #0 {
                  w323 = 50.0 ("y")
                  n184 = Add(x=w320, y=w323) -> (x+y=w322:dbl)
                  n185 = Add(x=w321, y=w323) -> (x+y=w324:dbl)
                  n186 = Build Array(w324, w322, 0.0 ("element")) -> (w315:dbl[])
                  n187 = local read "E727 error"() -> (w316:errorcluster)
                  n188 = local read "E727 Axes"() -> (w314:string[])
                  n189 = local read "E727"() -> (w319:i32)
                  n190 = property on="Cur_pos_x" class="DigNum (strict)"() -> ("Value"=w313:dbl)  [unwired: 2 in, 2 out]
                  n191 = property on="Cur_pos_y" class="DigNum (strict)"() -> ("Value"=w312:dbl)  [unwired: 2 in, 2 out]
                  n192 = call "MOV.vi"("System no."=w319, "Axes to move"=w314, "Position values"=w315, "error in"=w316) -> ("error out"=w308:errorcluster)  [unwired: 1 in, 14 out]
                  n193 = Add(x=w313, y=w312) -> (x+y=w311:dbl)
                  n194 = Equal?(x=w311, y=0.0) -> (x = y?=w309:bool)
                  n195 = case shown="True" w309 {
                    tunnel: w308 -> [w326 w327]
                    tunnel: [w326 w327] -> w307
                    frame False {
                    }
                    frame True {
                      n196 = Wait (ms)(milliseconds to wait=u32 500) -> ()  [unwired: 1 out]
                    }
                  }
                  n197 = call "POS?.vi"("System no."=w319, "All axes?"=TRUE, "error in"=w307) -> ()  [unwired: 2 in, 15 out]
                  n198 = Wait (ms)(milliseconds to wait=u32 20) -> ()  [unwired: 1 out]
                }
                frame #1 {
                  n199 = property on="LightField" class="LVClassControl (strict)"() -> (error out=w362:errorcluster, "Value"=w363:refnum<class "LightField Automation.lvclass">)  [unwired: 2 in, 1 out]
                  n200 = call "spec_getCalibration.vi"("error in (no error)"=w355, "LightField Automation in"=w363) -> ("error out"=w358:errorcluster, "ColumnCalibration"=w330:dbl[], "LightField Automation out"=w334:refnum<class "LightField Automation.lvclass">)  [unwired: 7 in]
                  n201 = Array Max & Min(array=w330) -> (max value=w351:dbl, min value=w350:dbl)  [unwired: 2 out]
                  n202 = Subtract(x=w351, y=w350) -> (x-y=w360:dbl)
                  n203 = local write "WL"(w330) -> ()
                  n204 = Divide(x=w360, y=2048.0) -> (x/y=w361:dbl)
                  n205 = property on="Pixel Information" class="IntGraph (strict)"(error in=w358, "XScale.Multiplier"=w361, "XScale.Offset"=w350) -> (error out=w359:errorcluster)  [unwired: 1 in, 1 out]
                  n206 = local read "map_data"() -> (w353:dbl[][][])
                  n207 = local read "Cur_pos_x"() -> (w345:dbl)
                  n208 = local read "Cur_pos_y"() -> (w344:dbl)
                  n209 = local read "i_min"() -> (w347:dbl)
                  n210 = local read "i_max"() -> (w349:dbl)
                  n211 = property on="Pixel Information" class="IntGraph (strict)"(error in=w359, "XScale.Maximum"=w351, "XScale.Minimum"=w350) -> (error out=w335:errorcluster)  [unwired: 1 in, 1 out]
                  n212 = property on="WL Slide" class="Slide (strict)"("Scale.Maximum"=w351, "Scale.Minimum"=w350) -> ()  [unwired: 2 in, 2 out]
                  n213 = local read "ROI"() -> (w329:i32)
                  n214 = call "LFA_Capture.vi"("error in (no error)"=w335, "LightField Automation in"=w334) -> ("error out"=w332:errorcluster, "Data"=w331:T3, "LightField Automation out"=w333:refnum<class "LightField Automation.lvclass">)  [unwired: 7 in]
                  n215 = call "Parse Data Object Simple.vi"("x"=w329, "Data"=w331) -> ("ROI 1, Frame 1, Row 1"=w348:dbl[], "ROI 1, Frame 1"=w357:dbl[][])  [unwired: 8 in]
                  n216 = Subtract(x=w349, y=w347) -> (x-y=w336:dbl)
                  n217 = Transpose 2D Array(2D array=w357) -> (transposed array=w354:dbl[][])
                  n218 = property on="LightField" class="LVClassControl (strict)"(error in=w362, "Value"=w333) -> ()  [unwired: 1 in, 2 out]
                  n219 = Replace Array Subset(array=w353, new element=w348, index (dim 0)=w345, index (dim 1)=w344) -> (w352:dbl[][][])  [unwired: 1 in]
                  n220 = Array Subset(array=w348, index=w347, length=w336) -> (w346:dbl[])
                  n221 = for {
                    tunnel: w352 -> [w374] mode=indexing
                    tunnel: [w373] -> w337 mode=indexing
                    tunnel: w336 -> [w372]
                    tunnel: w347 -> [w371]
                    n222 = for {
                      tunnel: w374 -> [w379] mode=indexing
                      tunnel: [w377] -> w373 mode=indexing
                      tunnel: w372 -> [w376]
                      tunnel: w371 -> [w375]
                      n223 = Array Subset(array=w379, index=w375, length=w376) -> (w378:dbl[])
                      n224 = Add Array Elements(numeric array=w378) -> (sum=w377:dbl)
                    }
                  }
                  n225 = Bundle("ColumnCalibration"=w330, "ROI 1, Frame 1, Row 1"=w348) -> (w364:T2)  [unwired: 1 in]
                  n226 = Add Array Elements(numeric array=w346) -> (sum=w340:dbl)
                  n227 = local write "PL spectrum"(w364) -> ()
                  n228 = Equal To 0?(x=w345) -> (x = 0?=w343:bool)
                  n229 = Equal To 0?(x=w344) -> (x = 0?=w342:bool)
                  n230 = And(x=w343, y=w342) -> (x .and. y?=w341:bool)
                  n231 = case shown="False" w341 {
                    tunnel: w340 -> [w369 w370]
                    tunnel: [w366 w370] -> w339
                    tunnel: [w365 w370] -> w338
                    frame False {
                      n232 = property on="map_plot" class="IntGraph (strict)"() -> ("ZScale.Maximum"=w368:dbl)  [unwired: 2 in, 2 out]
                      n233 = property on="map_plot" class="IntGraph (strict)"() -> ("ZScale.Minimum"=w367:dbl)  [unwired: 2 in, 2 out]
                      n234 = Max & Min(x=w369, y=w367) -> (min(x,y)=w366:dbl)  [unwired: 1 out]
                      n235 = Max & Min(x=w368, y=w369) -> (max(x,y)=w365:dbl)  [unwired: 1 out]
                    }
                    frame True {
                    }
                  }
                  n236 = local write "map_data"(w352) -> ()
                  n237 = local write "map_plot"(w337) -> ()
                  n238 = local write "Pixel Information"(w354) -> ()
                  n239 = property on="map_plot" class="IntGraph (strict)"("ZScale.Maximum"=w338) -> ()  [unwired: 2 in, 2 out]
                  n240 = property on="map_plot" class="IntGraph (strict)"("ZScale.Minimum"=w339) -> ()  [unwired: 2 in, 2 out]
                }
                frame #2 {
                  n241 = local read "WL"() -> (w393:dbl[])
                  n242 = local read "WL Slide"() -> (w384:cluster{dbl, dbl})
                  n243 = Unbundle(w384) -> (w381:dbl, w380:dbl)
                  n244 = Greater Or Equal?(x=w381, y=w380) -> (x >= y?=w395:bool)
                  n245 = Less?(x=w381, y=w380) -> (x < y?=w394:bool)
                  n246 = Select(t=w381, s=w394, f=w380) -> (s? t:f=w391:dbl)
                  n247 = Select(t=w381, s=w395, f=w380) -> (s? t:f=w392:dbl)
                  n248 = Array Max & Min(array=w393) -> (max value=w390:dbl, min value=w389:dbl)  [unwired: 2 out]
                  n249 = Threshold 1D Array(2:w392, 3:w393) -> (0:w387:dbl)  [unwired: 1 in]
                  n250 = Threshold 1D Array(2:w391, 3:w393) -> (0:w388:dbl)  [unwired: 1 in]
                  n251 = Round Toward -Infinity(1:w388) -> (0:w385:dbl)
                  n252 = Round Toward -Infinity(1:w387) -> (0:w386:dbl)
                  n253 = Increment(x=w386) -> (x+1=w383:dbl)
                  n254 = Increment(x=w385) -> (x+1=w382:dbl)
                  n255 = property on="WL Slide" class="Slide (strict)"("Scale.Maximum"=w390) -> ()  [unwired: 2 in, 2 out]
                  n256 = property on="WL Slide" class="Slide (strict)"("Scale.Minimum"=w389) -> ()  [unwired: 2 in, 2 out]
                  n257 = local write "i_min"(w382) -> ()
                  n258 = local write "i_max"(w383) -> ()
                }
                frame #3 {
                  n259 = case shown="\"increment\", Default" w401 {
                    tunnel: w400 -> [w404 w426]
                    tunnel: w399 -> [w403 w425]
                    tunnel: [w402 w428] -> w397
                    tunnel: [w407 w430] -> w398
                    tunnel: [w405 w427] -> w396
                    frame "decrement" {
                      n260 = local read "Min_x"() -> (w406:dbl)
                      n261 = Greater?(x=w404, y=w406) -> (0:w408:bool)
                      n262 = case shown="True" w408 {
                        tunnel: [enum16{"decrement", "increment"}."increment" ("Enum 2") enum16{"decrement", "increment"}."decrement" ("Enum 2")] -> w407
                        tunnel: w404 -> [w412 w422]
                        tunnel: [w415 w421] -> w405
                        tunnel: w403 -> [w414 w421]
                        tunnel: [w412 w420] -> w402
                        frame False {
                          n263 = property on="Cur_pos_y" class="DigNum (strict)"() -> (error out=w411:errorcluster, "Value"=w410:dbl)  [unwired: 2 in, 1 out]
                          n264 = local read "Step (um)"() -> (w413:dbl)
                          n265 = Add(x=w414, y=w413) -> (x+y=w415:dbl)
                          n266 = Increment(x=w410) -> (x+1=w409:dbl)
                          n267 = property on="Cur_pos_y" class="DigNum (strict)"(error in=w411, "Value"=w409) -> ()  [unwired: 1 in, 2 out]
                        }
                        frame True {
                          n268 = local read "Step (um)"() -> (w423:dbl)
                          n269 = property on="Cur_pos_x" class="DigNum (strict)"() -> (error out=w417:errorcluster, "Value"=w419:dbl)  [unwired: 2 in, 1 out]
                          n270 = Subtract(x=w422, y=w423) -> (x-y=w420:dbl)
                          n271 = Decrement(x=w419) -> (x-1=w418:dbl)
                          n272 = property on="Cur_pos_x" class="DigNum (strict)"(error in=w417, "Value"=w418) -> ()  [unwired: 1 in, 2 out]
                        }
                      }
                    }
                    frame "increment", Default {
                      n273 = local read "Max_x"() -> (w429:dbl)
                      n274 = Less?(x=w426, y=w429) -> (x < y?=w431:bool)
                      n275 = case shown="True" w431 {
                        tunnel: [enum16{"decrement", "increment"}."decrement" ("Enum 2") enum16{"decrement", "increment"}."increment" ("Enum 2")] -> w430
                        tunnel: w426 -> [w435 w445]
                        tunnel: [w435 w444] -> w428
                        tunnel: w425 -> [w437 w443]
                        tunnel: [w436 w443] -> w427
                        frame False {
                          n276 = local read "Step (um)"() -> (w438:dbl)
                          n277 = property on="Cur_pos_y" class="DigNum (strict)"() -> (error out=w432:errorcluster, "Value"=w434:dbl)  [unwired: 2 in, 1 out]
                          n278 = Add(x=w437, y=w438) -> (x+y=w436:dbl)
                          n279 = Increment(x=w434) -> (x+1=w433:dbl)
                          n280 = property on="Cur_pos_y" class="DigNum (strict)"(error in=w432, "Value"=w433) -> ()  [unwired: 1 in, 2 out]
                        }
                        frame True {
                          n281 = local read "Step (um)"() -> (w446:dbl)
                          n282 = property on="Cur_pos_x" class="DigNum (strict)"() -> (error out=w442:errorcluster, "Value"=w441:dbl)  [unwired: 2 in, 1 out]
                          n283 = Add(x=w445, y=w446) -> (x+y=w444:dbl)
                          n284 = Increment(x=w441) -> (x+1=w440:dbl)
                          n285 = property on="Cur_pos_x" class="DigNum (strict)"(error in=w442, "Value"=w440) -> ()  [unwired: 1 in, 2 out]
                        }
                      }
                    }
                  }
                }
              }
              n286 = local read "Total Count"() -> (w296:dbl)
              n287 = Increment(x=w292) -> (x+1=w297:i32)
              n288 = Wait (ms)(milliseconds to wait=u32 1) -> ()  [unwired: 1 out]
              n289 = Less?(x=w296, y=w297) -> (x < y?=w295:bool)
              n290 = Or(x=w295, y="2D Pause") -> (x .or. y?=w293:bool)
            }
            n291 = flat-sequence {
              tunnel: w261 -> [_]
              frame #0 {
                w291 = 50.0 ("y")
                n292 = local read "E727"() -> (w288:i32)
                n293 = local read "E727 Axes"() -> (w285:string[])
                n294 = Build Array(w291, w291, 0.0 ("element")) -> (w289:dbl[])
                n295 = local read "E727 error"() -> (w284:errorcluster)
                n296 = call "MOV.vi"("System no."=w288, "Axes to move"=w285, "Position values"=w289, "error in"=w284) -> ("error out"=w286:errorcluster)  [unwired: 1 in, 14 out]
                n297 = call "POS?.vi"("System no."=w288, "All axes?"=TRUE, "error in"=w286) -> ()  [unwired: 2 in, 15 out]
              }
            }
            "Cur_pos_x" <- w270
            "Cur_pos_y" <- w270
          }
          frame "Time-series save" {
            n298 = local read "Time-series graph"() -> (w455:dbl[][])
            n299 = local read "WL"() -> (w456:dbl[])
            n300 = local read "Time Interval (s)"() -> (w457:dbl)
            n301 = local read "Until when (s)"() -> (w462:dbl)
            n302 = Divide(x=w462, y=w457) -> (x/y=w461:dbl)
            n303 = for {
              N: w461 -> [_]
              tunnel: [w466] -> w450 mode=indexing
              tunnel: w457 -> [w465]
              i -> [w464]
              n304 = Multiply(x=w465, y=w464) -> (x*y=w466:dbl)
            }
            n305 = Insert Into Array(array=w455, index (col)=0 ("index (row)"), new element=w456) -> (w454:dbl[][])  [unwired: 1 in]
            n306 = Insert Into Array(array=w450, index=0, new element=0.0 ("new element/subarray")) -> (w449:dbl[])
            n307 = Insert Into Array(array=w454, index (row)=0 ("disabled index (col)"), new element=w449) -> (w458:dbl[][])  [unwired: 1 in]
            n308 = call-poly <vilib>:"Write Delimited Spreadsheet.vi"("2D data"=w458) -> ("error out"=w460:errorcluster)  [unwired: 13 in, 1 out]
            n309 = call <vilib>:"Clear Errors.vi"("error in (no error)"=w460, "specific error code to clear (0: all)"=43) -> ()  [unwired: 4 in, 2 out]
          }
          frame "Load" {
            w490 = u16 2 items=["RS232", "TCP/IP", "USB"] ("Interface")
            n310 = Path To String(path=path "C:/Users/localAdmin/Documents/test/SDK 1.2.4 Installer/SDK 1.2.4 Installer/M000010157.xml") -> (string=w472:string)
            n311 = call "PE Create.vi"("error in (no error)"=w474, "conffile"=w472) -> ("error out"=w477:errorcluster, "peHandle"=w467:u64)  [unwired: 8 in]
            "LLTF port" <- w467
            n312 = call "LFA_Initialize.vi"("error in (no error)"=w474) -> ("error out"=w495:errorcluster, "LightField Automation out"=w494:refnum<class "LightField Automation.lvclass">)  [unwired: 9 in]
            n313 = local read "E727"() -> (w479:i32)
            n314 = call "PE Get System Name.vi"("error in (no error)"=w477, "index"=0, "peHandle"=w467) -> ("error out"=w476:errorcluster, "name"=w468:string)  [unwired: 7 in]
            "Current system" <- w468
            n315 = call "PE Open.vi"("error in (no error)"=w476, "name"=w468, "peHandle"=w467) -> ("error out"=w475:errorcluster)  [unwired: 8 in]
            n316 = call "Exp_SetExperiment.vi"("error in (no error)"=w495, "ExperimentName"="Experiment name", "LightField Automation in"=w494) -> ("error out"=w491:errorcluster, "LightField Automation out"=w492:refnum<class "LightField Automation.lvclass">)  [unwired: 7 in]
            n317 = call "E727_Configuration_Setup.vi"("System no."=w479, "USB settings"="USB settings", "error in"=w474, "Interface"=w490, "Timeout"=u32 5000) -> ("error out"=w488:errorcluster)  [unwired: 9 in, 5 out]
            n318 = call "PE Get Wavelength Range.vi"("error in (no error)"=w475, "peHandle"=w467) -> ("error out"=w473:errorcluster, "maximum"=→"Max Wavelength":dbl, "minimum"=→"Min Wavelength":dbl)  [unwired: 7 in]
            "LLTF error" <- w473
            n319 = call "Define connected axes.vi"("System no."=w479, "Read from\ncontroller?"=TRUE ("Read from\ncontroller?"), "Invert\norder?"=FALSE ("Invert\norder?"), "error in"=w488) -> ("Conn. Axes out"=w483:string[], "error out"=w487:errorcluster)  [unwired: 1 in, 13 out]
            "E727 Axes" <- w483
            n320 = property on="LightField" class="LVClassControl (strict)"(error in=w491, "Value"=w492) -> (error out=w482:errorcluster)  [unwired: 1 in, 1 out]
            n321 = call "CST?.vi"("System no."=w479, "Axes to query"=w483, "error in"=w487) -> ("error out"=w481:errorcluster)  [unwired: 2 in, 14 out]
            "E727 error" <- w481
            n322 = Merge Errors(w482, w481, w473) -> (w480:errorcluster)
          }
        }
      }
      frame Error {
      }
    }
  }
  n323 = while {
    shift-right: [w500] -> w5
    shift-left: w7 -> [w503]
    shift-right: [w501] -> w6
    shift-left: w8 -> [w502]
    stop <- w498 stop-if-true
    # "Producer"
    n324 = event shown="[10] \"Load\": Value Change" {
      selector: _ -> [_ _ _ _ _ _ _ _ _ _ _ _ _ _ _]
      dyn-events: _ -> [_ _ _ _ _ _ _ _ _ _ _ _ _ _ _]
      timeout: _ -> [_ _ _ _ _ _ _ _ _ _ _ _ _ _ _]
      tunnel: w503 -> [w506 w509 w515 w529 w561 w573 w579 w584 w589 w594 w599 w604 w609 w614 w620]
      tunnel: [w506 w507 w513 w529 w561 w572 w577 w582 w587 w593 w597 w602 w607 w612 w617] -> w500
      tunnel: w502 -> [w505 w510 w516 w530 w562 w574 w580 w585 w590 w595 w600 w605 w610 w615 w619]
      tunnel: [w505 w508 w514 w530 w562 w571 w578 w583 w588 w592 w598 w603 w608 w613 w618] -> w501
      tunnel: [_ _ "stop" _ _ _ _ _ _ _ _ _ _ _ _] -> w499
      event Timeout {
        n325 = event-data() -> ()  [unwired: 1 in, 3 out]
      }
      event "Single Acquire": Value Change {
        n326 = event-data() -> ()  [unwired: 1 in, 6 out]
        n327 = Enqueue Element(queue=w510, element="Single Acquire", error in (no error)=w509) -> (queue out=w508:refnum<queue>, error out=w507:errorcluster)  [unwired: 1 in, 1 out]
      }
      event "stop": Value Change {
        n328 = event-data() -> ()  [unwired: 1 in, 1 out]
        n329 = Enqueue Element(queue=w516, element="Stop", error in (no error)=w515) -> (queue out=w514:refnum<queue>, error out=w513:errorcluster)  [unwired: 1 in, 1 out]
      }
      event "WL Slide": Value Change {
        n330 = event-data() -> ("NewVal"=w527:cluster{dbl, dbl})  [unwired: 1 in]
        n331 = Unbundle(w527) -> (w547:dbl, w544:dbl)
        n332 = Unbundle(w527) -> (w526:dbl, w525:dbl)
        n333 = property on="WL Slide" class="Slide (strict)"() -> ("Active Slider"=w523:i32)  [unwired: 2 in, 2 out]
        n334 = Less Or Equal?(x=w526, y=w525) -> (x <= y?=w524:bool)
        n335 = Greater Or Equal?(x=w547, y=w544) -> (x >= y?=w546:bool)
        n336 = Less?(x=w547, y=w544) -> (x < y?=w545:bool)
        n337 = case shown="True" w524 {
          tunnel: w523 -> [w549 w550]
          tunnel: [w549 w550] -> w520
          tunnel: [3 ("Active Slider") 4 ("Active Slider")] -> w518
          frame False {
          }
          frame True {
          }
        }
        n338 = local read "WL"() -> (w535:dbl[])
        n339 = Select(t=w547, s=w546, f=w544) -> (s? t:f=w543:dbl)
        n340 = Select(t=w547, s=w545, f=w544) -> (s? t:f=w542:dbl)
        n341 = Threshold 1D Array(2:w543, 3:w535) -> (0:w540:dbl)  [unwired: 1 in]
        n342 = Threshold 1D Array(2:w542, 3:w535) -> (0:w541:dbl)  [unwired: 1 in]
        n343 = Array Max & Min(array=w535) -> (max value=w537:dbl, min value=w536:dbl)  [unwired: 2 out]
        n344 = Round Toward -Infinity(1:w541) -> (0:w538:dbl)
        n345 = Round Toward -Infinity(1:w540) -> (0:w539:dbl)
        n346 = Increment(x=w538) -> (x+1=w532:dbl)
        "i_min" <- w532
        n347 = Increment(x=w539) -> (x+1=w534:dbl)
        "i_max" <- w534
        n348 = property on="WL Slide" class="Slide (strict)"("Active Slider"=0) -> (error out=w521:errorcluster)  [unwired: 2 in, 1 out]
        n349 = property on="WL Slide" class="Slide (strict)"("Scale.Minimum"=w536) -> ()  [unwired: 2 in, 2 out]
        n350 = property on="WL Slide" class="Slide (strict)"("Scale.Maximum"=w537) -> ()  [unwired: 2 in, 2 out]
        n351 = Subtract(x=w534, y=w532) -> (x-y=w533:dbl)
        n352 = property on="WL Slide" class="Slide (strict)"(error in=w521, "Fill Style"=w518) -> (error out=w519:errorcluster)  [unwired: 1 in, 1 out]
        n353 = property on="WL Slide" class="Slide (strict)"(error in=w519, "Active Slider"=w520) -> ()  [unwired: 1 in, 2 out]
        n354 = local read "map_data"() -> (w531:dbl[][][])
        n355 = for {
          tunnel: w531 -> [w555] mode=indexing
          tunnel: [w554] -> w528 mode=indexing
          tunnel: w533 -> [w553]
          tunnel: w532 -> [w552]
          n356 = for {
            tunnel: w555 -> [w560] mode=indexing
            tunnel: [w558] -> w554 mode=indexing
            tunnel: w553 -> [w557]
            tunnel: w552 -> [w556]
            n357 = Array Subset(array=w560, index=w556, length=w557) -> (w559:dbl[])
            n358 = Add Array Elements(numeric array=w559) -> (sum=w558:dbl)
          }
        }
        n359 = local write "map_plot"(w528) -> ()
      }
      event "map_plot": Cursor Move {
        n360 = event-data() -> ("CursLoc"=w569:cluster{"X":dbl, "Y":dbl})  [unwired: 1 in, 8 out]
        n361 = Unbundle(w569) -> ("X"=w567:dbl, "Y"=w566:dbl)
        n362 = local read "map_data"() -> (w568:dbl[][][])
        n363 = Index Array(array=w568, index (dim 0)=w567, index (dim 1)=w566) -> (element=w564:dbl[])  [unwired: 1 in]
        n364 = local read "WL"() -> (w565:dbl[])
        n365 = Bundle("WL"=w565, "map_data"=w564) -> (w563:cluster{"WL":dbl[], "map_data":dbl[]})  [unwired: 1 in]
        n366 = local write "PL spectrum"(w563) -> ()
      }
      event "2D map_save": Value Change {
        n367 = event-data() -> ()  [unwired: 1 in, 6 out]
        n368 = Enqueue Element(queue=w574, element="2D map_save", error in (no error)=w573) -> (queue out=w571:refnum<queue>, error out=w572:errorcluster)  [unwired: 1 in, 1 out]
      }
      event "Time-series": Value Change {
        n369 = event-data() -> ()  [unwired: 1 in, 6 out]
        n370 = Enqueue Element(queue=w580, element="Time-series", error in (no error)=w579) -> (queue out=w578:refnum<queue>, error out=w577:errorcluster)  [unwired: 1 in, 1 out]
        "Time-counting" <- 0.0 ("Time-counting")
      }
      event "Time-series save": Value Change {
        n371 = event-data() -> ()  [unwired: 1 in, 6 out]
        n372 = Enqueue Element(queue=w585, element="Time-series save", error in (no error)=w584) -> (queue out=w583:refnum<queue>, error out=w582:errorcluster)  [unwired: 1 in, 1 out]
      }
      event "PLE start": Value Change {
        n373 = event-data() -> ()  [unwired: 1 in, 6 out]
        n374 = Enqueue Element(queue=w590, element="PLE start", error in (no error)=w589) -> (queue out=w588:refnum<queue>, error out=w587:errorcluster)  [unwired: 1 in, 1 out]
      }
      event "PLE save": Value Change {
        n375 = event-data() -> ()  [unwired: 1 in, 6 out]
        n376 = Enqueue Element(queue=w595, element="PLE save", error in (no error)=w594) -> (queue out=w592:refnum<queue>, error out=w593:errorcluster)  [unwired: 1 in, 1 out]
      }
      event "Load": Value Change {
        n377 = event-data() -> ()  [unwired: 1 in, 1 out]
        n378 = Enqueue Element(queue=w600, element="Load", error in (no error)=w599) -> (queue out=w598:refnum<queue>, error out=w597:errorcluster)  [unwired: 1 in, 1 out]
      }
      event "2D map": Value Change {
        n379 = event-data() -> ()  [unwired: 1 in, 1 out]
        n380 = Enqueue Element(queue=w605, element="2D map", error in (no error)=w604) -> (queue out=w603:refnum<queue>, error out=w602:errorcluster)  [unwired: 1 in, 1 out]
      }
      event "Centre WL (nm)": Value Change {
        n381 = event-data() -> ()  [unwired: 1 in, 1 out]
        n382 = Enqueue Element(queue=w610, element="Centre WL", error in (no error)=w609) -> (queue out=w608:refnum<queue>, error out=w607:errorcluster)  [unwired: 1 in, 1 out]
      }
      event "Exposure Time (ms)": Value Change {
        n383 = event-data() -> ()  [unwired: 1 in, 6 out]
        n384 = Enqueue Element(queue=w615, element="Exposure Time", error in (no error)=w614) -> (queue out=w613:refnum<queue>, error out=w612:errorcluster)  [unwired: 1 in, 1 out]
      }
      event "Laser WL (nm)": Value Change {
        n385 = event-data() -> ()  [unwired: 1 in, 6 out]
        n386 = Enqueue Element(queue=w619, element="Laser Wavelength", error in (no error)=w620) -> (queue out=w618:refnum<queue>, error out=w617:errorcluster)  [unwired: 1 in, 1 out]
      }
    }
    n387 = Wait (ms)(milliseconds to wait=u32 1) -> ()  [unwired: 1 out]
    n388 = Or(x=w500, y=w499) -> (x .or. y?=w498:bool)
  }
  n389 = Release Queue(queue=w6, error in (no error)=w5) -> (error out=w3:errorcluster)  [unwired: 1 in, 2 out]
  n390 = Merge Errors(w3, w2) -> (→"error out":errorcluster)
